vi "Power Guard Example.vi"() -> ()   [LabVIEW 2012, in "Phidget Power Guard.lvlib"]
uses:
  <instrlib>/Phidgets/Phidget Power Guard/Phidget Power Guard.lvlib
  <instrlib>/Phidgets/Phidget Power Guard/Public/PowerGuardStart.vi
  <instrlib>/Phidgets/Phidget Power Guard/Public/PowerGuardClose.vi
  <instrlib>/Phidgets/Phidget Common/Phidget Common.lvlib
panel:
  in  "Enabled":bool
  in  "Fan Mode":u32(ring)=3 items=["FAN_MODE_OFF"=1, "FAN_MODE_ON"=2, "FAN_MODE_AUTO"=3]
  in  "Over Voltage":dbl=-1.0
  out "error out":errorcluster
  in  "error in (no error)":errorcluster
  in  "Device Info":T1={"Serial Number"=-1, "Channel"=0, "Port"=0}
  out "Attached?":bool
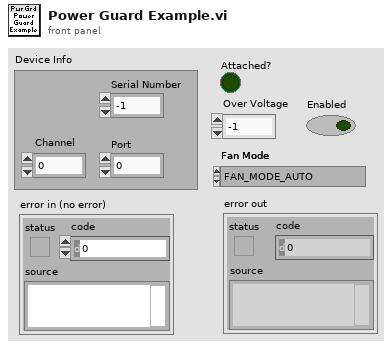
[diagram p1: front panel]
types:
  T1 = cluster{"Serial Number":i32, "Channel":i32, "Port":i32}
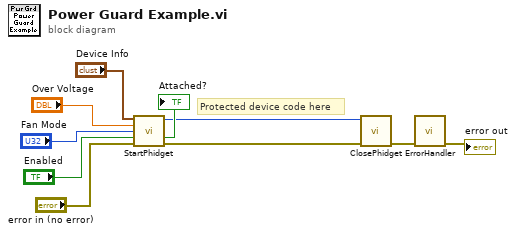
[diagram p0: block diagram]
diagram:
  # "Protected device code here"
  n1 = call-poly <instrlib>:"StartPhidget.vi"("Device Info"="Device Info", "Over Voltage"="Over Voltage", "Fan Mode"="Fan Mode", "Enabled"="Enabled", "error in (no error)"="error in (no error)") -> ("Phidget ID"=w2:u64, "Attached?"=→"Attached?":bool, "error out"=w1:errorcluster)  [unwired: 7 in, 1 out]
  n2 = call-poly <instrlib>:"ClosePhidget.vi"("error in"=w1, "Device In"=w2) -> ("error out"=w7:errorcluster)  [unwired: 9 in]
  n3 = call <instrlib>:"ErrorHandler.vi"("error in"=w7) -> ("error out"=→"error out":errorcluster)  [unwired: 9 in, 1 out]
